vi "WMI Get Brightness.vi"() -> ()   [LabVIEW 2012]
uses:
  System.Management
panel:
  in  "error out":errorcluster
  out "error out":errorcluster
  out "ToString":string
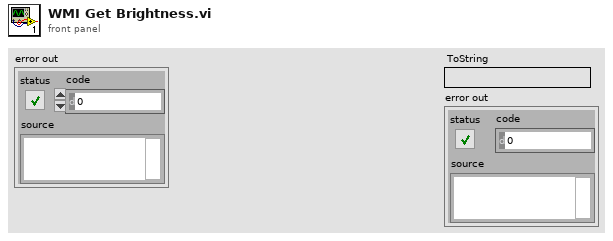
[diagram p1: front panel]
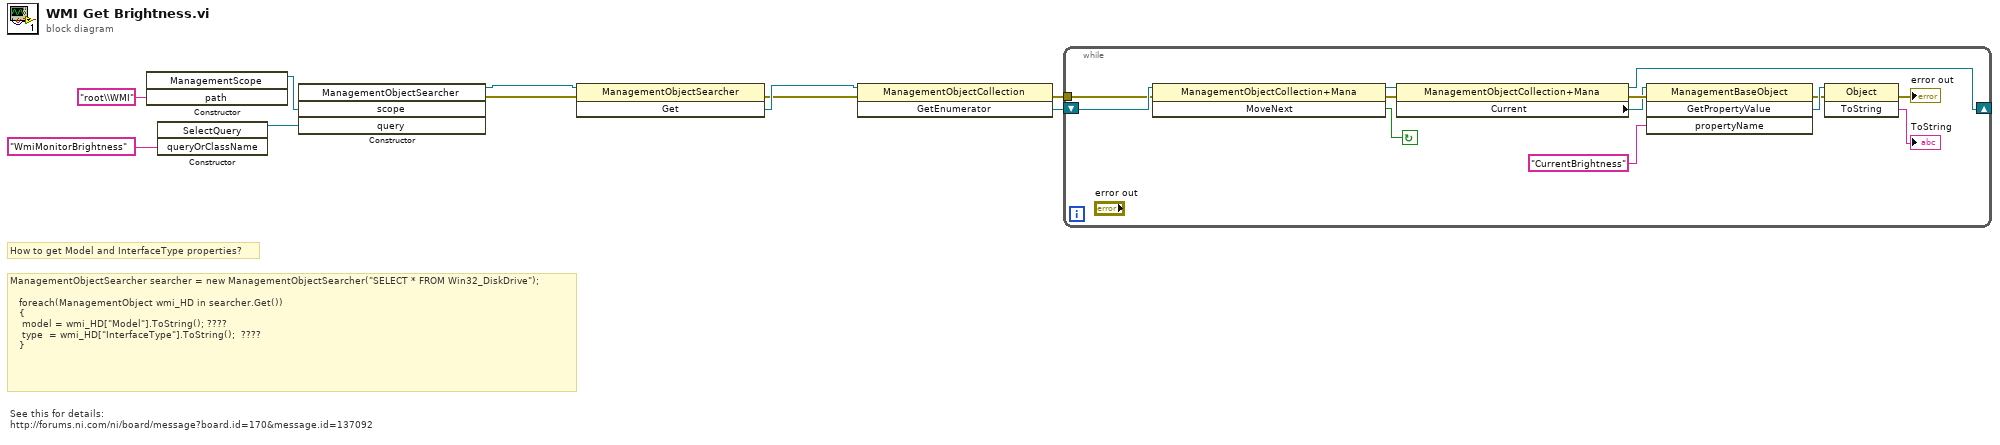
[diagram p0: block diagram]
diagram:
  # "See this for details: \nhttp://forums.ni.com/ni/board/message?board.id=170&message.id=137092"
  # "How to get Model and InterfaceType properties?"
  # "ManagementObjectSearcher searcher = new ManagementObjectSearcher(\"SELECT * FROM Win32_DiskDrive\");\n\n   foreach(ManagementObject wmi_HD in searcher.Get())\n   {\n    model = wmi_HD[\"Model\"].ToString(); ????\n    type  = wmi_HD[\"InterfaceType\"].ToString();  ????\n   }"
  n1 = constructor class="ManagementScope"("path"="root\\WMI") -> (reference out=w3:refnum<k24>)  [unwired: 3 in, 3 out]
  n2 = constructor class="SelectQuery"("queryOrClassName"="WmiMonitorBrightness") -> (reference out=w1:refnum<k24>)  [unwired: 3 in, 3 out]
  n3 = constructor class="ManagementObjectSearcher"("scope"=w3, "query"=w1) -> (reference out=w10:refnum<k24>, error out=w6:errorcluster)  [unwired: 3 in, 3 out]
  n4 = invoke class="ManagementObjectSearcher" method="Get"(reference=w10, error in=w6) -> (error out=w5:errorcluster, "Get"=w9:refnum<k24>)  [unwired: 1 in, 1 out]
  n5 = invoke class="ManagementObjectCollection" method="GetEnumerator"(reference=w9, error in=w5) -> (error out=w8:errorcluster, "GetEnumerator"=w7:refnum<k24>)  [unwired: 1 in, 1 out]
  n6 = while {
    shift-right: [w13] -> _
    shift-left: w7 -> [w18]
    tunnel: w8 -> [w11]
    stop <- w17 continue-if-true
    n7 = invoke class="ManagementObjectCollection+Mana" method="MoveNext"(reference=w18, error in=w11) -> (reference out=w16:refnum<k24>, error out=w15:errorcluster, "MoveNext"=w17:bool)  [unwired: 1 in]
    n8 = property class="ManagementObjectCollection+Mana"(reference=w16, error in=w15) -> (reference out=w13:refnum<k24>, error out=w21:errorcluster, "Current"=w19:refnum<k24>)
    n9 = invoke class="ManagementBaseObject" method="GetPropertyValue"(reference=w19, error in=w21, "propertyName"="CurrentBrightness") -> (error out=w14:errorcluster, "GetPropertyValue"=w22:refnum<k24>)  [unwired: 1 in, 2 out]
    n10 = invoke class="Object" method="ToString"(reference=w22, error in=w14) -> (error out=→"error out":errorcluster, "ToString"=→"ToString":string)  [unwired: 1 in, 1 out]
  }
